vi "Set Body.vi"(8 "error in (no error)":errorcluster, 10 "Body":string, 11 "Gmail in":refnum<class "Gmail.lvclass">) -> (0 "error out":errorcluster, 3 "Gmail out":refnum<class "Gmail.lvclass">)   [LabVIEW 2020, in "Gmail API.lvlib" / "Gmail.lvclass"]
doc: "Sets the content of the email. This can be HTML or plaintext. If sending HTML email content, ensure that the Content-Type property is set to \"text/html\"."
uses:
  Gmail.lvclass
  Gmail.lvclass/Gmail.ctl
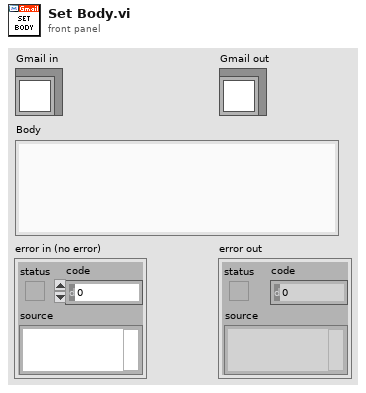
[diagram p1: front panel]
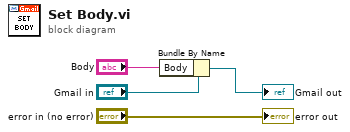
[diagram p0: block diagram]
diagram:
  n1 = Bundle By Name(cluster="Gmail in", "Body"="Body") -> (→"Gmail out":refnum<class "Gmail.lvclass">)
  "error out" <- "error in (no error)"
